vi "fpga_status.vi"(8 "error in (no error)":errorcluster, 11 "USRP_1_x_200MHz in":refnum<class "USRP_1_x_200MHz.lvclass">) -> (0 "error out":errorcluster, 2 "pulse TX status":T1, 3 "USRP_1_x_200MHz out":refnum<class "USRP_1_x_200MHz.lvclass">)   [LabVIEW 2021, in "USRP_1_x_200MHz.lvclass"]
uses:
  USRP_1_x_200MHz.lvclass
  USRP_1_x_200MHz.lvclass/USRP_1_x_200MHz.ctl
  <vilib>/Utility/error.llb/Error Cluster From Error Code.vi
  <vilib>/rvi/errors/niLvFpgaAdjustHostInterfaceError.vi
  <vilib>/rvi/interface/nirviReadWriteControl/nirviReadWriteControl.xnode
  NiFpgaLv.dll
  <vilib>/rvi/interface/Simulation/niFpgaSimulationCallBeginRW.vi
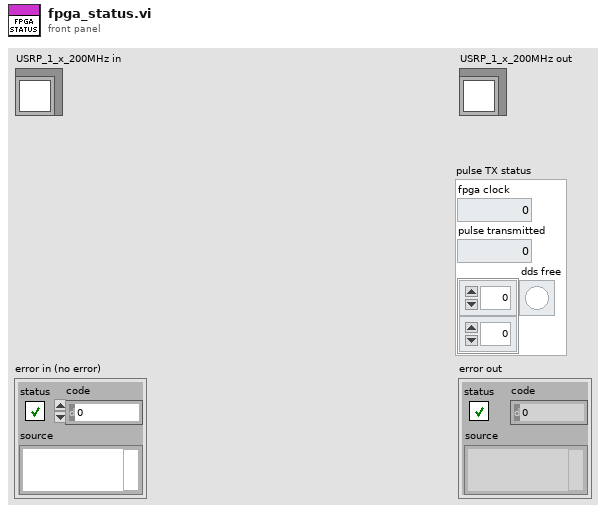
[diagram p1: front panel]
types:
  T1 = cluster{"fpga clock":dbl, "pulse transmitted":u32, "dds free":bool[][]}
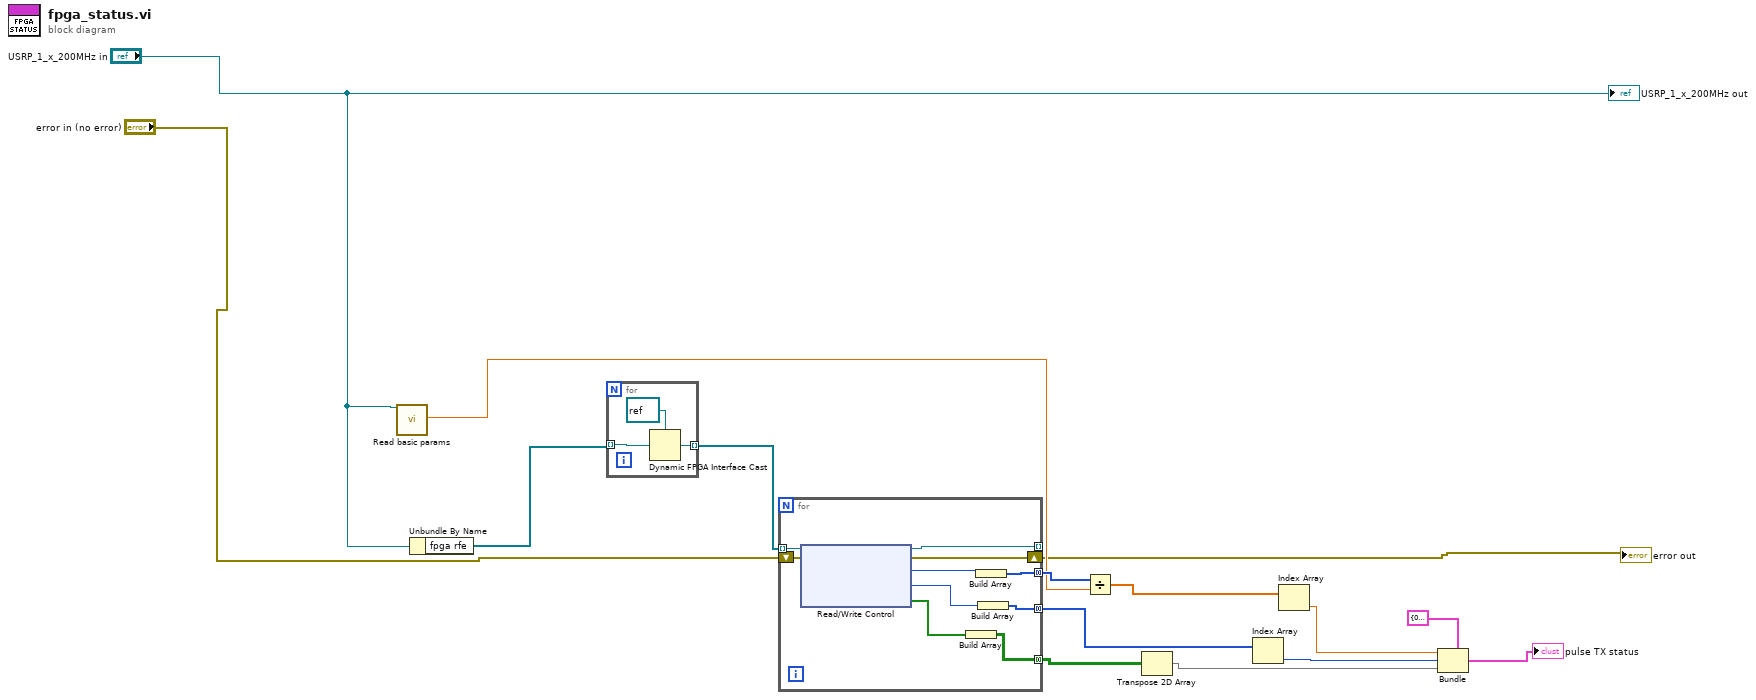
[diagram p0: block diagram]
diagram:
  n1 = call-dynamic "Read basic params.vi"("device_type in"="USRP_1_x_200MHz in") -> ("Fs  FPGA"=w11:dbl)  [unwired: 13 in, 5 out]
  n2 = Unbundle By Name("USRP_1_x_200MHz in") -> ("fpga rfe"=w13:refnum<k20>[])
  n3 = for {
    tunnel: w13 -> [w18] mode=indexing
    tunnel: [w16] -> w14 mode=indexing
    n4 = Dynamic FPGA Interface Cast(Session In=refnum<k20> refnum ("fpga interface out"), Type=w18) -> (Session Out=w16:refnum<k20>)
  }
  n5 = for {
    tunnel: w14 -> [w25] mode=indexing
    shift-right: [w27] -> w3
    shift-left: "error in (no error)" -> [w28]
    tunnel: [w26] -> _ mode=indexing
    tunnel: [w23] -> w12 mode=concatenating
    tunnel: [w21] -> w6 mode=concatenating
    tunnel: [w19] -> w15 mode=concatenating
    n6 = xnode "Read/Write Control"("FPGA VI Reference In"=w25, "error in"=w28) -> ("FPGA VI Reference Out"=w26:refnum<k20>, "error out"=w27:errorcluster, "fpga clock"=w20:u64, "pulse transmitted"=w22:u32, "dds free"=w24:bool[])
    n7 = Build Array(w24) -> (w23:bool[][])
    n8 = Build Array(w20) -> (w19:u64[])
    n9 = Build Array(w22) -> (w21:u32[])
  }
  "error out" <- w3
  n10 = Divide(x=w15, y=w11) -> (x/y=w8:dbl[])
  n11 = Transpose 2D Array(2D array=w12) -> (transposed array=w9:bool[][])
  n12 = Index Array(array=w6) -> (element=w5:u32)  [unwired: 1 in]
  n13 = Index Array(array=w8) -> (element=w7:dbl)  [unwired: 1 in]
  n14 = Bundle(cluster=T1 {"fpga clock"=0.0, "pulse transmitted"=0, "dds free"=[[FALSE, FALSE, FALSE, FALSE, FALSE, FALSE, FALSE, FALSE, FALSE, FALSE, FALSE, FALSE, FALSE, FALSE, FALSE, FALSE]]} ("pulse TX status"), "fpga clock"=w7, "pulse transmitted"=w5, "dds free"=w9) -> (→"pulse TX status":T1)
  "USRP_1_x_200MHz out" <- "USRP_1_x_200MHz in"
